vi "Write cost.vi"(8 "error in (no error)":errorcluster, 10 "price":dbl, 11 "Furniture in":refnum<class "Furniture.lvclass">) -> (0 "error out":errorcluster, 3 "Furniture out":refnum<class "Furniture.lvclass">)   [LabVIEW 2021, in "Furniture.lvclass"]
uses:
  Furniture.lvclass
  Furniture.lvclass/Furniture.ctl
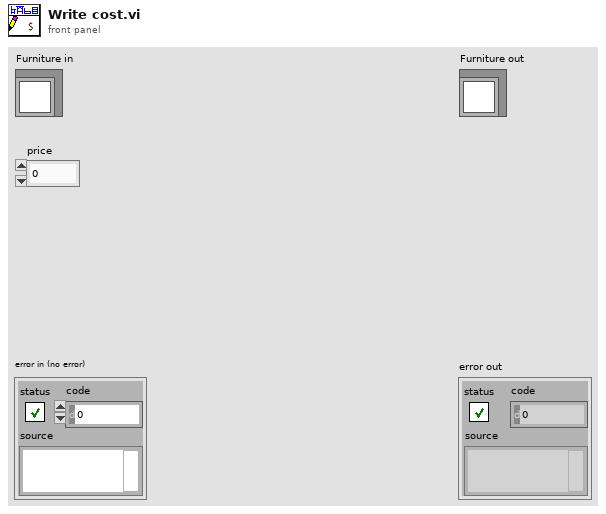
[diagram p1: front panel]
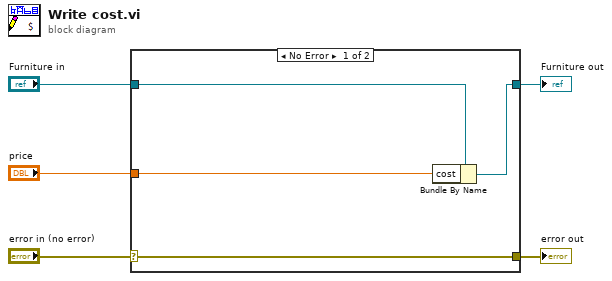
[diagram p0: block diagram]
diagram:
  n1 = case shown="No Error" "error in (no error)" {
    selector: "error in (no error)" -> [w9 w10]
    tunnel: [w9 w10] -> w4
    tunnel: [w7 w11] -> w2
    tunnel: "Furniture in" -> [w8 w11]
    tunnel: "price" -> [w6 _]
    frame No Error {
      n2 = Bundle By Name(cluster=w8, "cost"=w6) -> (w7:refnum<class "Furniture.lvclass">)
    }
    frame Error {
    }
  }
  "error out" <- w4
  "Furniture out" <- w2
